vi "Handle Mouse Down.vi"(4 "PlatMods":T1, 5 "VolatusAPI":refnum<class "VolatusAPI.lvclass">, 6 "Mods":cluster{"Double Click":bool, "Menu Key":bool}, 7 "CtlRef":refnum<vi>, 8 "error in (no error)":errorcluster, 9 "Coords":T2, 10 "Button":u16, 11 "DigitalButtonControl in":refnum<class "DigitalButtonControl.lvclass">) -> (0 "error out":errorcluster, 3 "DigitalButtonControl out":refnum<class "DigitalButtonControl.lvclass">)   [LabVIEW 2020, in "VolatusGUIElements.lvlib" / "DigitalButtonControl.lvclass"]
uses:
  DigitalButtonControl.lvclass
  <vilib>/Utility/miscctls.llb/LVPoint32TypeDef.ctl
  Volatus/VolatusAPI/VolatusAPI.lvclass
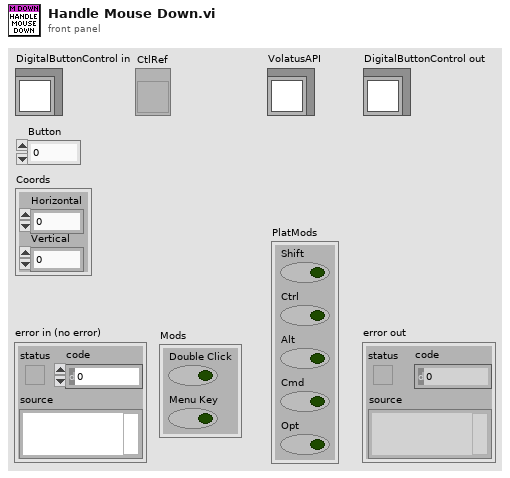
[diagram p1: front panel]
types:
  T1 = cluster{"Shift":bool, "Ctrl":bool, "Alt":bool, "Cmd":bool, "Opt":bool}
  T2 = typedef "LVPoint32TypeDef.ctl" = cluster{"Horizontal":i32, "Vertical":i32}
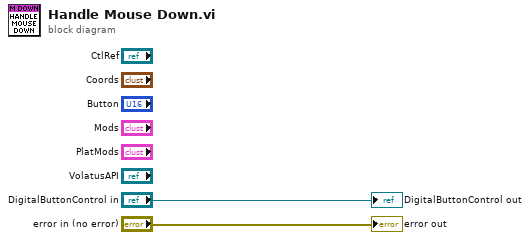
[diagram p0: block diagram]
diagram:
  "error out" <- "error in (no error)"
  "DigitalButtonControl out" <- "DigitalButtonControl in"
